vi "BT DUT Update Type.vi"(8 "error in (no error)":errorcluster, 11 "niDTS BT DUT in":refnum<class "niDTS BT Dut.lvclass">) -> (0 "error out":errorcluster, 3 "niDTS BT DUT out":refnum<class "niDTS BT Dut.lvclass">)   [LabVIEW 2015, in "niDTS BT.lvlib" / "niDTS BT Dut.lvclass"]
doc: "Updates the WLAN Type according to changes made individually to Standard, Rate, or Streams."
uses:
  niDTS BT Dut.lvclass
  niDTS BT Dut.lvclass/niDTS BT Dut.ctl
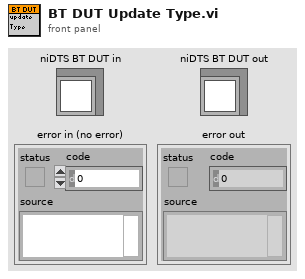
[diagram p1: front panel]
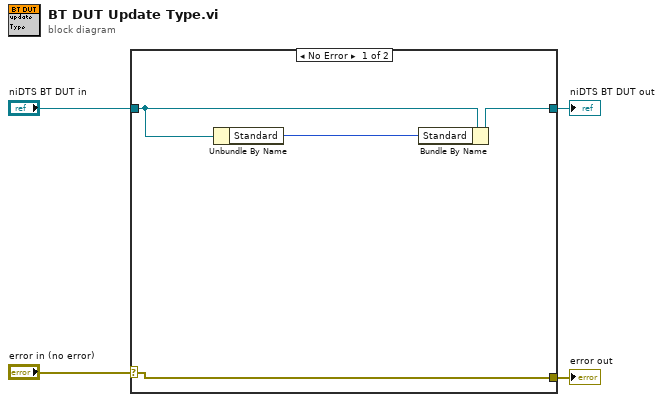
[diagram p0: block diagram]
diagram:
  n1 = case shown="No Error" "error in (no error)" {
    selector: "error in (no error)" -> [w6 w10]
    tunnel: [w6 w10] -> w3
    tunnel: [w7 w9] -> w1
    tunnel: "niDTS BT DUT in" -> [w8 w9]
    frame No Error {
      n2 = Unbundle By Name(w8) -> ("Standard"=w5:enum16{"BDR", "EDR", "LE"})
      n3 = Bundle By Name(cluster=w8, "Standard"=w5) -> (w7:refnum<class "niDTS BT Dut.lvclass">)
    }
    frame Error {
    }
  }
  "error out" <- w3
  "niDTS BT DUT out" <- w1
